vi "sv_Compute Combinations of Intermodulation Coefficients.vi"(10 "maximum order":u8=3, 11 "number of tones":i32=10) -> (3 "intermodulation coefficients":cluster{"order":i32, "digit array":u8[][]}[](array[cluster]))   [LabVIEW 2017]
doc: "Use this VI to compute intermodulation (mix) combinations (M*f1 +/- N*f2 ... +/- P*fmax) up to specified maximum order where order is sum(M,N,...,P)."
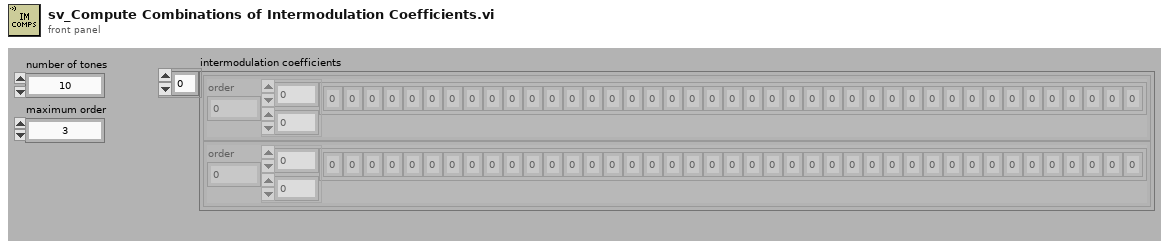
[diagram p1: front panel]
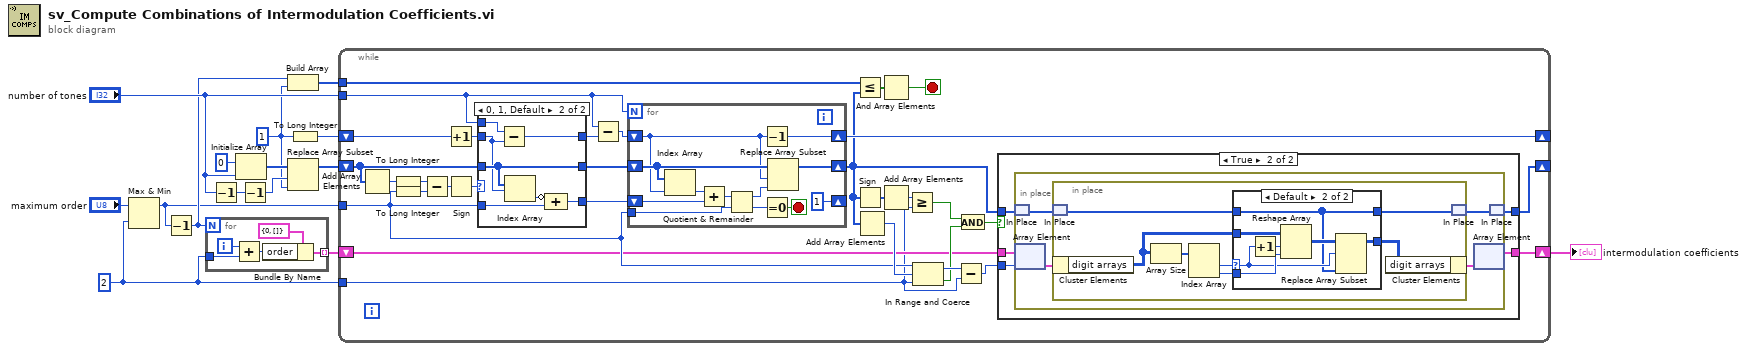
[diagram p0: block diagram]
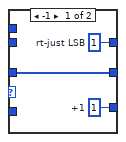
[diagram p2: hidden frame]
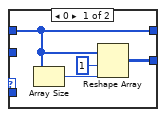
[diagram p4: hidden frame]
diagram:
  w1 = u8 2 ("x")
  w4 = u8 1 ("new element/subarray")
  n1 = Max & Min(x="maximum order", y=w1) -> (max(x,y)=w2:u8)  [unwired: 1 out]
  n2 = Decrement(x=w2) -> (x-1=w7:u8)
  n3 = for {
    N: w7 -> [_]
    tunnel: [w19] -> w13 mode=indexing
    tunnel: w1 -> [w17]
    i -> [w20]
    n4 = Add(x=w20, y=w17) -> (x+y=w18:i32)
    n5 = Bundle By Name(cluster=cluster{"order":i32, "digit arrays":u8[][]} {"order"=0, "digit arrays"=[]}, "order"=w18) -> (w19:cluster{"order":i32, "digit arrays":u8[][]})
  }
  n6 = Decrement(x="number of tones") -> (x-1=w6:i32)
  n7 = Initialize Array(u8 0 ("order"), "number of tones") -> (w11:u8[])
  n8 = Decrement(x=w6) -> (x-1=w9:i32)
  n9 = Build Array(w7, w4) -> (w8:u8[])
  n10 = Replace Array Subset(array=w11, new element=w4, index=w9) -> (w10:u8[])
  n11 = To Long Integer(number=w4) -> (32bit integer=w5:i32)
  n12 = while {
    shift-right: [w26] -> _
    shift-left: w10 -> [w33]
    tunnel: w2 -> [w27]
    shift-right: [w37] -> w14
    shift-left: w13 -> [w23]
    tunnel: "number of tones" -> [w29]
    tunnel: w8 -> [w43]
    tunnel: w1 -> [w22]
    shift-right: [w30] -> _
    shift-left: w5 -> [w25]
    stop <- w35 stop-if-true
    n13 = Add Array Elements(numeric array=w33) -> (sum=w42:u8)
    n14 = To Long Integer(number=w42) -> (32bit integer=w38:i32)
    n15 = To Long Integer(number=w27) -> (32bit integer=w36:i32)
    n16 = Subtract(x=w38, y=w36) -> (x-y=w41:i32)
    n17 = Increment(x=w25) -> (x+1=w24:i32)
    n18 = Sign(1:w41) -> (0:w39:i32)
    n19 = case shown="0, 1, Default" w39 {
      tunnel: [w54 w61] -> w32
      tunnel: w33 -> [w54 w61]
      tunnel: [w53 w56] -> w34
      tunnel: [w52 w57] -> w31
      tunnel: w29 -> [_ w60]
      tunnel: w27 -> [_ w59]
      tunnel: w24 -> [_ w55]
      frame -1 {
        w52 = u8 1  # +1
        w53 = 1  # rt-just LSB
      }
      frame 0, 1, Default {
        n20 = Subtract(x=w60, y=w55) -> (x-y=w56:i32)
        n21 = Index Array(array=w61, index=w55) -> (element=w58:u8)
        n22 = Compound Arithmetic op=ADD(invert w58, w59) -> (w57:u8)
      }
    }
    n23 = Subtract(x=w29, y=w34) -> (x-y=w40:i32)
    n24 = for {
      N: w29 -> [_]
      shift-right: [w69] -> w30
      shift-left: w40 -> [w66]
      shift-right: [w68] -> w21
      shift-left: w32 -> [w67]
      tunnel: w27 -> [w72]
      shift-right: [u8 1 ("initial increment")] -> _
      shift-left: w31 -> [w62]
      stop <- w71 stop-if-true
      n25 = Index Array(array=w67, index=w66) -> (element=w65:u8)
      n26 = Add(x=w65, y=w62) -> (x+y=w73:u8)
      n27 = Quotient & Remainder(x=w73, y=w72) -> (x-y*floor(x/y)=w64:u8, floor(x/y)=w70:u8)
      n28 = Decrement(x=w66) -> (x-1=w69:i32)
      n29 = Equal To 0?(x=w70) -> (x = 0?=w71:bool)
      n30 = Replace Array Subset(array=w67, new element=w64, index=w66) -> (w68:u8[])
    }
    n31 = Less Or Equal?(x=w43, y=w21) -> (x <= y?=w51:bool[])
    n32 = Sign(1:w21) -> (0:w46:u8[])
    n33 = Add Array Elements(numeric array=w21) -> (sum=w48:u8)
    n34 = And Array Elements(Boolean array=w51) -> (logical AND=w35:bool)
    n35 = Add Array Elements(numeric array=w46) -> (sum=w45:u8)
    n36 = Greater Or Equal?(x=w45, y=w22) -> (x >= y?=w50:bool)
    n37 = In Range and Coerce(upper limit=w27, x=w48, lower limit=w22) -> (coerced(x)=w47:u8, In Range?=w44:bool)
    n38 = Subtract(x=w47, y=w22) -> (x-y=w28:u8)
    n39 = And(x=w50, y=w44) -> (x .and. y?=w49:bool)
    n40 = case shown="True" w49 {
      tunnel: w23 -> [w75 w80]
      tunnel: w21 -> [w74 w77]
      tunnel: [w75 w79] -> w37
      tunnel: w28 -> [_ w78]
      tunnel: [w74 w76] -> w26
      frame False {
      }
      frame True {
        n41 = in-place {
          n42 = in-place-match #1(w77) -> (w82:u8[])
          n43 = in-place-array #2(w80, w78) -> (w84:cluster{"order":i32, "digit arrays":u8[][]})
          n44 = in-place {
            n45 = in-place-match #3(w82) -> (w89:u8[])
            n46 = in-place-cluster #4(w84) -> ("digit arrays"=w87:u8[][])
            n47 = Array Size(array=w87) -> (size(s)=w91:i32[])
            n48 = Index Array(array=w91) -> (element #1=w86:i32, element #2=w90:i32)  [unwired: 2 in]
            n49 = case shown="Default" w86 {
              selector: w86 -> [_ w97]
              tunnel: w90 -> [_ w101]
              tunnel: w89 -> [w92 w96]
              tunnel: [w93 w99] -> w88
              tunnel: w87 -> [_ w98]
              tunnel: [w92 w96] -> w85
              frame 0 {
                n50 = Array Size(array=w92) -> (size(s)=w94:i32)
                n51 = Reshape Array(w92, 1 ("dimension size"), w94) -> (w93:u8[][])
              }
              frame Default {
                n52 = Increment(x=w97) -> (x+1=w102:i32)
                n53 = Reshape Array(w98, w102, w101) -> (w100:u8[][])
                n54 = Replace Array Subset(array=w100, new element=w96, index (row)=w97) -> (w99:u8[][])  [unwired: 1 in]
              }
            }
            n55 = in-place-cluster #4("digit arrays"=w88) -> (w83:cluster{"order":i32, "digit arrays":u8[][]})
            n56 = in-place-match #3(w85) -> (w81:u8[])
          }
          n57 = in-place-array #2(w83) -> (w79:cluster{"order":i32, "digit arrays":u8[][]}[])  [unwired: 1 out]
          n58 = in-place-match #1(w81) -> (w76:u8[])
        }
      }
    }
  }
  "intermodulation coefficients" <- w14
